vi "Configure Trigger Model.vi"(0 "VISA resource name":refnum<visa-resource-name>, 1 "Buffer Name (defbuffer1)":string="defbuffer1", 2 "Number of Times to repeat (1)":i32=1 format="%#.6g", 3 "Timer Interval (1us)":dbl=5e-05 min=5e-05 max=10000.0, 4 "Trigger Count (1)":i32=1 format="%#.6g", 5 "error in (no error)":errorcluster, 6 "Trigger Delay (1 us)":dbl=5e-05 min=5e-05 max=10000.0) -> (14 "VISA resource name out":refnum<visa-resource-name>, 19 "error out":errorcluster)   [LabVIEW 2018, in "Keithley 2450.lvlib"]
doc: "Configures the trigger model similar to 2400 model."
uses:
  <instrlib>/Keithley 2450/Keithley 2450.lvlib
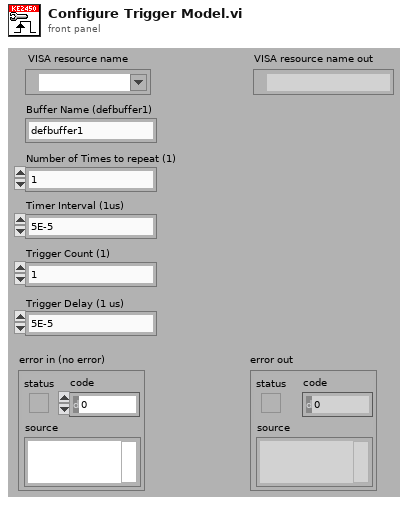
[diagram p1: front panel]
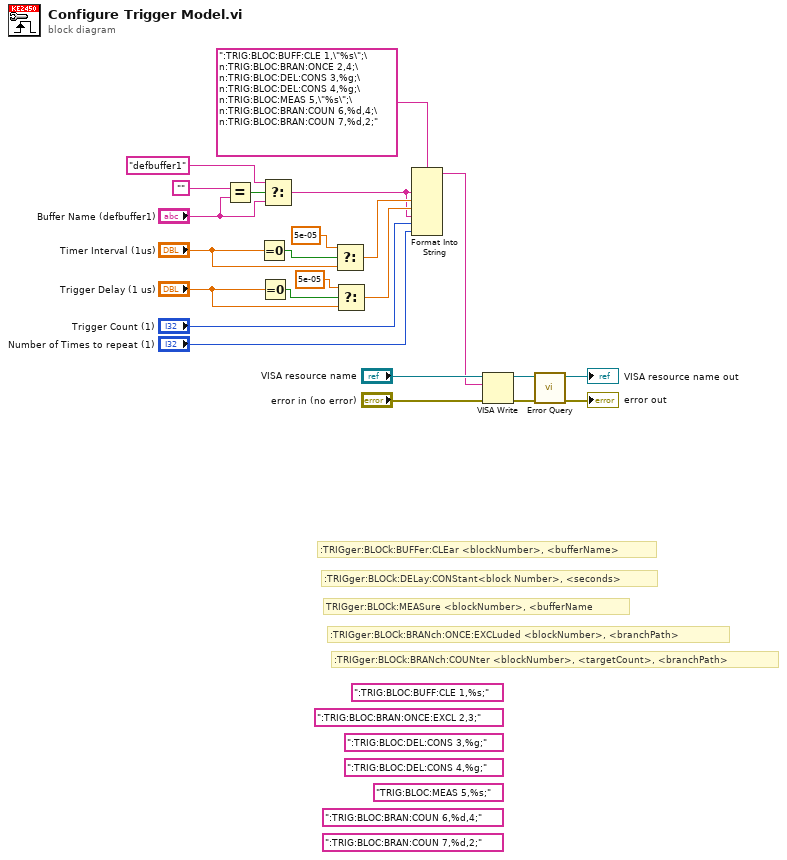
[diagram p0: block diagram]
diagram:
  (unwired) ":TRIG:BLOC:BRAN:COUN 7,%d,2;"
  (unwired) ":TRIG:BLOC:BRAN:COUN 6,%d,4;"
  (unwired) "TRIG:BLOC:MEAS 5,%s;"
  (unwired) ":TRIG:BLOC:DEL:CONS 4,%g;"
  (unwired) ":TRIG:BLOC:DEL:CONS 3,%g;"
  (unwired) ":TRIG:BLOC:BRAN:ONCE:EXCL 2,3;"
  (unwired) ":TRIG:BLOC:BUFF:CLE 1,%s;"
  # ":TRIGger:BLOCk:BRANch:COUNter <blockNumber>, <targetCount>, <branchPath>"
  # ":TRIGger:BLOCk:BRANch:ONCE:EXCLuded <blockNumber>, <branchPath>"
  # "TRIGger:BLOCk:MEASure <blockNumber>, <bufferName"
  # ":TRIGger:BLOCk:DELay:CONStant<block Number>, <seconds>"
  # ":TRIGger:BLOCk:BUFFer:CLEar <blockNumber>, <bufferName>"
  n1 = Equal?(x="", y="Buffer Name (defbuffer1)") -> (x = y?=w8:bool)
  n2 = Equal To 0?(x="Timer Interval (1us)") -> (x = 0?=w17:bool)
  n3 = Equal To 0?(x="Trigger Delay (1 us)") -> (x = 0?=w13:bool)
  n4 = Select(t="defbuffer1", s=w8, f="Buffer Name (defbuffer1)") -> (s? t:f=w5:string)
  n5 = Select(t=5e-05, s=w17, f="Timer Interval (1us)") -> (s? t:f=w14:dbl)
  n6 = Select(t=5e-05, s=w13, f="Trigger Delay (1 us)") -> (s? t:f=w10:dbl)
  n7 = Format Into String(format string=":TRIG:BLOC:BUFF:CLE 1,\"%s\";\n:TRIG:BLOC:BRAN:ONCE 2,4;\n:TRIG:BLOC:DEL:CONS 3,%g;\n:TRIG:BLOC:DEL:CONS 4,%g;\n:TRIG:BLOC:MEAS 5,\"%s\";\n:TRIG:BLOC:BRAN:COUN 6,%d,4;\n:TRIG:BLOC:BRAN:COUN 7,%d,2;", w5, w14, w10, w5, "Trigger Count (1)", "Number of Times to repeat (1)") -> (resulting string=w18:string)  [unwired: 2 in, 1 out]
  n8 = VISA Write(VISA resource name="VISA resource name", write buffer=w18, error in (no error)="error in (no error)") -> (VISA resource name out=w2:refnum<visa-resource-name>, error out=w4:errorcluster)  [unwired: 1 out]
  n9 = call <instrlib>:"Error Query.vi"("error in (no error)"=w4, "VISA resource name"=w2) -> ("error out"=→"error out":errorcluster, "VISA resource name out"=→"VISA resource name out":refnum<visa-resource-name>)  [unwired: 8 out]
